vi "DiffDrivePoseEst2_InterpRecord_Interp.vi"(6 "Extra":variant, 9 "Time Fraction":dbl, 10 "End Input 2":variant, 11 "Input 1":variant) -> (3 "Interp Output":variant)   [LabVIEW 2019, in "Trajectory_Library.lvlib"]
uses:
  Trajectory_Library.lvlib
  TypeDef/TRANSLATION2D.ctl
  TypeDef/ROTATION2D.ctl
  TypeDef/POSE2D.ctl
  TypeDef/DIFF_DRIVE_POSE_EST2_INTERP_RECORD.ctl
  TypeDef/DIFF_DRIVE_KINEMATICS.ctl
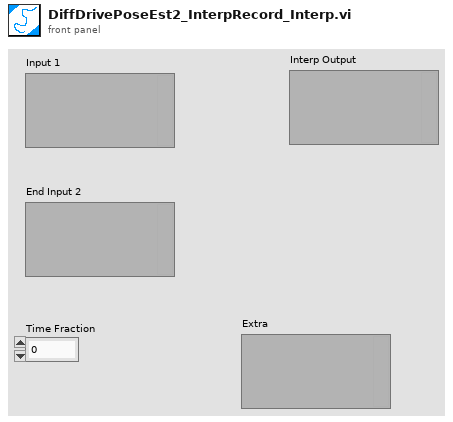
[diagram p1: front panel]
types:
  T1 = typedef "Trajectory_Library.lvlib/DIFF_DRIVE_POSE_EST2_INTERP_RECORD.ctl" = cluster{"PoseMeters":T2, "GyroAngle":T4, "LeftMeters":dbl, "RightMeters":dbl}
  T2 = typedef "Trajectory_Library.lvlib/POSE2D.ctl" = cluster{"TRANSLATION":T3, "ROTATION":T4}
  T3 = typedef "Trajectory_Library.lvlib/TRANSLATION2D.ctl" = cluster{"X":dbl, "Y":dbl}
  T4 = typedef "Trajectory_Library.lvlib/ROTATION2D.ctl" = cluster{"VALUE":dbl, "COS":dbl, "SIN":dbl}
  T5 = typedef "Trajectory_Library.lvlib/DIFF_DRIVE_KINEMATICS.ctl" = cluster{"TrackWidth_Meters":dbl}
  T6 = typedef "Trajectory_Library.lvlib/TWIST2D.ctl" = cluster{"dX":dbl, "dY":dbl, "dTHETA":dbl}
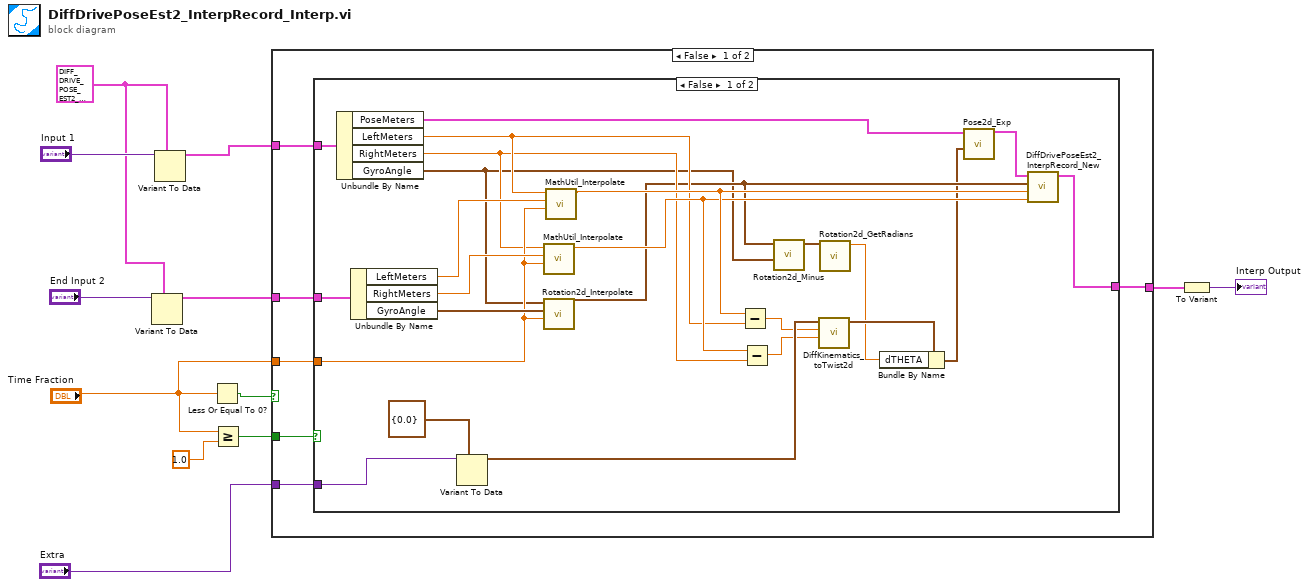
[diagram p0: block diagram]
diagram:
  w10 = T1 {"PoseMeters"={"TRANSLATION"={"X"=0.0, "Y"=0.0}, "ROTATION"={"VALUE"=0.0, "COS"=1.0, "SIN"=0.0}}, "GyroAngle"={"VALUE"=0.0, "COS"=1.0, "SIN"=0.0}, "LeftMeters"=0.0, "RightMeters"=0.0} ("DIFF_DRIVE_POSE_EST2_INTERP_RECORD")
  n1 = Variant To Data(type=w10, Variant="End Input 2") -> (data=w3:T1)  [unwired: 1 in, 1 out]
  n2 = Variant To Data(type=w10, Variant="Input 1") -> (data=w8:T1)  [unwired: 1 in, 1 out]
  n3 = Less Or Equal To 0?(x="Time Fraction") -> (x <= 0?=w9:bool)
  n4 = Greater Or Equal?(x="Time Fraction", y=1.0) -> (x >= y?=w4:bool)
  n5 = case shown="False" w9 {
    tunnel: [w17 w44] -> w6
    tunnel: w8 -> [w15 w44]
    tunnel: w4 -> [w18 _]
    tunnel: w3 -> [w16 _]
    tunnel: "Time Fraction" -> [w14 _]
    tunnel: "Extra" -> [w13 _]
    frame False {
      n6 = case shown="False" w18 {
        tunnel: [w19 w43] -> w17
        tunnel: w16 -> [w41 w43]
        tunnel: w15 -> [w42 _]
        tunnel: w14 -> [w37 _]
        tunnel: w13 -> [w36 _]
        frame False {
          n7 = Unbundle By Name(w42) -> ("PoseMeters"=w22:T2, "LeftMeters"=w32:dbl, "RightMeters"=w31:dbl, "GyroAngle"=w25:T4)
          n8 = Unbundle By Name(w41) -> ("LeftMeters"=w40:dbl, "RightMeters"=w39:dbl, "GyroAngle"=w38:T4)
          n9 = Variant To Data(type=T5 {"TrackWidth_Meters"=0.0} ("DIFF_DRIVE_KINEMATICS"), Variant=w36) -> (data=w30:T5)  [unwired: 1 in, 1 out]
          n10 = call "MathUtil_Interpolate.vi"("T"=w37, "EndValue"=w39, "StartValue"=w31) -> ("InterpolatedValue"=w33:dbl)  [unwired: 8 in]
          n11 = call "Rotation2d_Interpolate.vi"("T"=w37, "EncValue ROTATION"=w38, "in ROTATION"=w25) -> ("Interpolated ROTATION"=w26:T4)  [unwired: 8 in]
          n12 = call "MathUtil_Interpolate.vi"("T"=w37, "EndValue"=w40, "StartValue"=w32) -> ("InterpolatedValue"=w34:dbl)  [unwired: 8 in]
          n13 = Subtract(x=w34, y=w32) -> (x-y=w29:dbl)
          n14 = Subtract(x=w33, y=w31) -> (x-y=w28:dbl)
          n15 = call "Rotation2d_Minus.vi"("other ROTATION"=w25, "in ROTATION"=w26) -> ("out ROTATION"=w24:T4)  [unwired: 9 in]
          n16 = call "DiffKinematics_toTwist2d.vi"("Right Distance M"=w28, "Left Distance M"=w29, "DIFF_DRIVE_KINEMATICS"=w30) -> ("Twist2d"=w27:T6)  [unwired: 8 in]
          n17 = call "Rotation2d_GetRadians.vi"("in ROTATION"=w24) -> ("AngleRadians"=w23:dbl)  [unwired: 10 in]
          n18 = Bundle By Name(cluster=w27, "dTHETA"=w23) -> (w20:T6)
          n19 = call "Pose2d_Exp.vi"("TWIST"=w20, "POSE"=w22) -> ("UpdatedPose"=w21:T2)  [unwired: 9 in]
          n20 = call "DiffDrivePoseEst2_InterpRecord_New.vi"("RightDistance"=w33, "LeftDistance"=w34, "GyroAngle"=w26, "M_POSE_Meters"=w21) -> ("DIFF_DRIVE_POSE_EST2_INTERP_RECORD"=w19:T1)  [unwired: 7 in]
        }
        frame True {
        }
      }
    }
    frame True {
    }
  }
  n21 = To Variant(anything=w6) -> (Variant=→"Interp Output":variant)
